vi "Get DataArray.vi"(8 "error in (no error)":errorcluster, 11 "DataTable in":refnum<class "DataTable.lvclass">) -> (0 "error out":errorcluster, 2 "Array":variant[][](array[variant]), 3 "DataTable out":refnum<class "DataTable.lvclass">)   [LabVIEW 2013, in "DataGrid.lvlib" / "DataTable.lvclass"]
uses:
  DataTable.lvclass
  DataTable.lvclass/DataTable.ctl
  System.Data
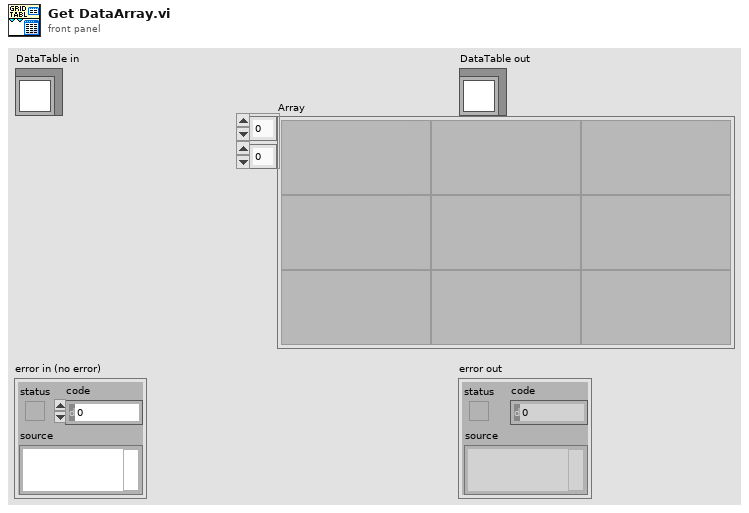
[diagram p1: front panel]
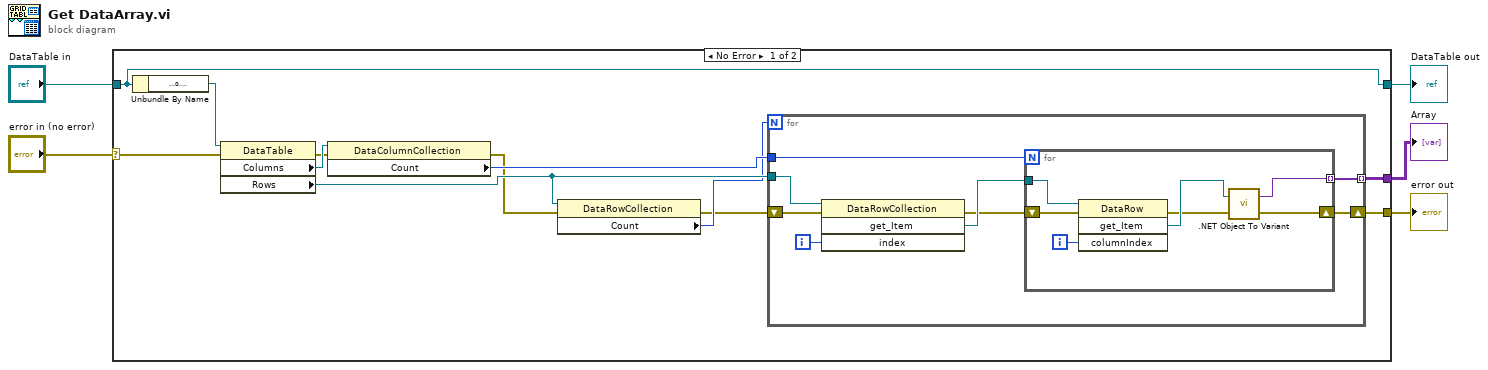
[diagram p0: block diagram]
diagram:
  n1 = case shown="No Error" "error in (no error)" {
    selector: "error in (no error)" -> [w10 w33]
    tunnel: [w9 w33] -> w4
    tunnel: [w17 w34] -> w2
    tunnel: "DataTable in" -> [w17 w34]
    tunnel: [w8 _] -> w1
    frame No Error {
      n2 = Unbundle By Name(w17) -> ("DataTable"=w16:refnum<k24>)
      n3 = property class="DataTable"(reference=w16, error in=w10) -> (error out=w11:errorcluster, "Columns"=w15:refnum<k24>, "Rows"=w13:refnum<k24>)  [unwired: 1 out]
      n4 = property class="DataColumnCollection"(reference=w15, error in=w11) -> (error out=w7:errorcluster, "Count"=w14:i32)  [unwired: 1 out]
      n5 = property class="DataRowCollection"(reference=w13, error in=w7) -> (error out=w6:errorcluster, "Count"=w12:i32)  [unwired: 1 out]
      n6 = for {
        N: w12 -> [_]
        tunnel: w14 -> [w25]
        tunnel: w13 -> [w24]
        shift-right: [w21] -> w9
        shift-left: w6 -> [w20]
        tunnel: [w19] -> w8 mode=indexing
        i -> [w23]
        n7 = invoke class="DataRowCollection" method="get_Item"(reference=w24, error in=w20, "index"=w23) -> (error out=w18:errorcluster, "get_Item"=w22:refnum<k24>)  [unwired: 1 in, 2 out]
        n8 = for {
          N: w25 -> [_]
          tunnel: w22 -> [w32]
          shift-right: [w26] -> w21
          shift-left: w18 -> [w30]
          tunnel: [w29] -> w19 mode=indexing
          i -> [w31]
          n9 = invoke class="DataRow" method="get_Item"(reference=w32, error in=w30, "columnIndex"=w31) -> (error out=w27:errorcluster, "get_Item"=w28:refnum<k24>)  [unwired: 1 in, 2 out]
          n10 = call <vilib>:".NET Object To Variant.vi"("error in (no error)"=w27, ".NET object"=w28) -> ("error out"=w26:errorcluster, "variant"=w29:variant)
        }
      }
    }
    frame Error {
    }
  }
  "error out" <- w4
  "DataTable out" <- w2
  "Array" <- w1
